vi "example_llm_azureopenai_unit_test_1.vi"() -> ()   [LabVIEW 2020]
uses:
  src/models/llm_azureopenai_chatmodels/llm_azureopenai_chatmodels.lvclass
  src/models/message_text/message_text.lvclass
  D:/lv_llm/labview-llm-libraries/src/models/abstract_message_base/abstract_message_base.lvclass
  src/models/message_text/message.ctl
panel:
  out "azureopenai_url":string
  in  "Messages":cluster{"role":string, "text":string}[](array[cluster])=[{"role"="system", "text"="Act as a math teacher and guide the student in solving the problem. You should not solve the problem. Always answer in single line."}, {"role"="user", "text"="What is x in the equation 2x + 3 = 5  ?"}]
  out "error out":errorcluster
  out "azureopenai_key":string
  in  "deployement name":string(combo)="gpt-4o-mini"
  # "1. Ensure you assign the Azure OpenAI Key & URL to environmental variables so it is away from the code and easy to use the examples in future.\n\n2. Use the \"Set_Env_Var.vi\" from examples/utils folder to set the key \"labview_llm_azureopenai_key\" and \"labview_llm_azureopenai_url\"."
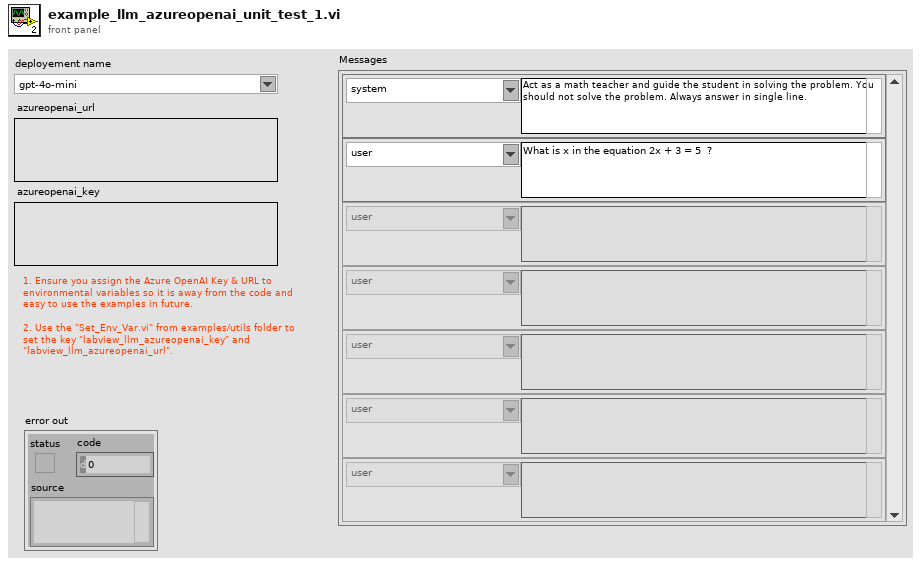
[diagram p1: front panel]
types:
  T1 = typedef "message_text.lvclass/message.ctl" = cluster{"role":string, "content":string[]}
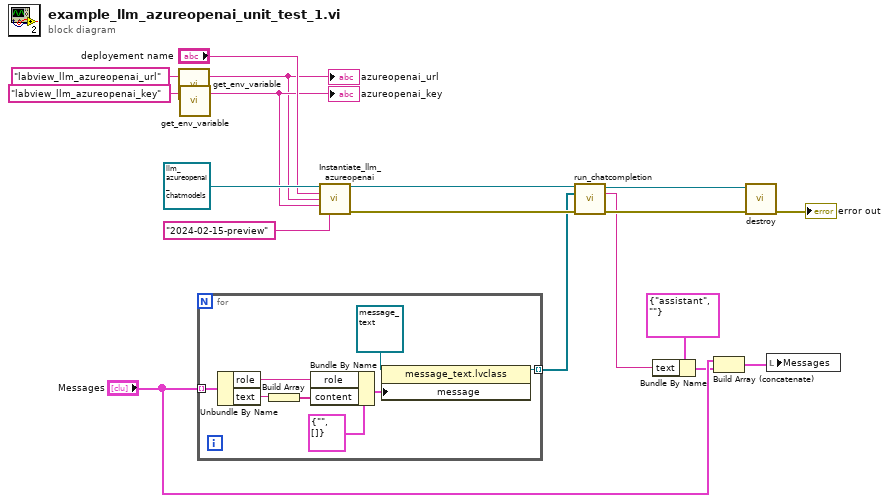
[diagram p0: block diagram]
diagram:
  n1 = call "get_env_variable.vi"("Environment Variable Name"="labview_llm_azureopenai_url") -> ("Value"=w1:string)  [unwired: 1 in, 1 out]
  "azureopenai_url" <- w1
  n2 = call "get_env_variable.vi"("Environment Variable Name"="labview_llm_azureopenai_key") -> ("Value"=w2:string)  [unwired: 1 in, 1 out]
  "azureopenai_key" <- w2
  n3 = for {
    tunnel: "Messages" -> [w24] mode=indexing
    tunnel: [w25] -> w12 mode=indexing
    n4 = Unbundle By Name(w24) -> ("role"=w22:string, "text"=w20:string)
    n5 = Build Array(w20) -> (w19:string[])
    n6 = Bundle By Name(cluster=T1 {"role"="", "content"=[]} ("message"), "role"=w22, "content"=w19) -> (w21:T1)
    n7 = property class="message_text.lvclass"(reference=refnum<class "message_text.lvclass"> refnum ("message_text.lvclass"), "message"=w21) -> (reference out=w25:refnum<class "message_text.lvclass">)  [unwired: 1 in, 1 out]
  }
  n8 = call "Instantiate_llm_azureopenai.vi"("llm_azureopenai_chatmodels in"=refnum<class "llm_azureopenai_chatmodels.lvclass"> refnum ("llm_openai in"), "deployement name"="deployement name", "azure_endpoint"=w1, "azure_api_key"=w2, "api_version"="2024-02-15-preview") -> ("llm_azureopenai_chatmodels out"=w18:refnum<class "llm_azureopenai_chatmodels.lvclass">, "error out"=w17:errorcluster)  [unwired: 9 in]
  n9 = call-dynamic "run_chatcompletion.vi"("chatcompletion_llm_interface in"=w18, "Messages"=w12, "error in (no error)"=w17) -> ("chatcompletion_llm_interface out"=w15:refnum<class "llm_azureopenai_chatmodels.lvclass">, "chat response"=w8:string, "error out"=w14:errorcluster)  [unwired: 10 in]
  n10 = Bundle By Name(cluster=cluster{"role":string, "text":string} {"role"="assistant", "text"=""} ("message"), "text"=w8) -> (w7:cluster{"role":string, "text":string})
  n11 = Build Array (concatenate)("Messages", w7) -> (w10:cluster{"role":string, "text":string}[])
  n12 = call-dynamic "destroy.vi"("error in (no error)"=w14, "abstract_llm_base in"=w15) -> ("error out"=→"error out":errorcluster)  [unwired: 8 in, 1 out]
  n13 = local write "Messages"(w10) -> ()
